vi "Pair Nodes.vi"(8 "error in (no error)":errorcluster, 10 "Node UID to Pair":string, 11 "E2E editor node in":refnum<data-value>) -> (0 "error out":errorcluster, 3 "E2E editor node out":refnum<data-value>)   [LabVIEW 2015, in "E2E Tag Exchange editor node.lvclass"]
uses:
  E2E Tag Exchange editor node.lvclass
  Node LUT/Command.ctl
  Node LUT/Node LUT.lvlib
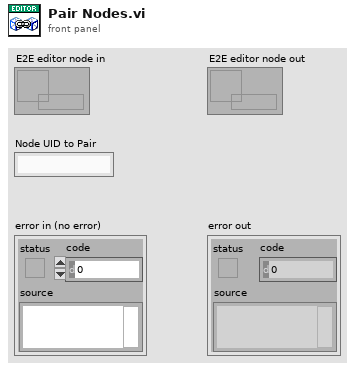
[diagram p1: front panel]
types:
  T1 = typedef "Node LUT.lvlib/Command.ctl" = enum16{"Initialize", "Add Node", "Remove Node", "Node Ref from UID", "List Nodes"}
  T2 = typedef "NISE_CEF_Node.lvclass/NodeRef.ctl" = refnum<data-value>
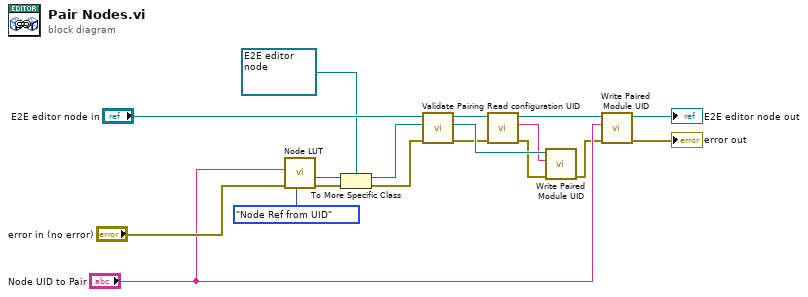
[diagram p0: block diagram]
diagram:
  n1 = call "Node LUT.vi"("Command"=Command."Node Ref from UID", "error in"="error in (no error)", "UID"="Node UID to Pair") -> ("error out"=w14:errorcluster, "node ref"=w15:T2)  [unwired: 5 in, 2 out]
  n2 = To More Specific Class(target class=refnum<data-value> refnum, reference=w15, error in=w14) -> (specific class reference=w12:refnum<data-value>, error out=w11:errorcluster)
  n3 = call "Validate Pairing.vi"("error in (no error)"=w11, "E2E node 2"=w12, "E2E node 1"="E2E editor node in") -> ("error out"=w4:errorcluster, "E2E node 2 out"=w5:refnum<data-value>, "E2E node 1 out"=w7:refnum<data-value>)  [unwired: 6 in]
  n4 = call "Read configuration UID.vi"("error in (no error)"=w4, "E2E editor node in"=w7) -> ("error out"=w3:errorcluster, "Module UID"=w2:string, "E2E editor node out"=w6:refnum<data-value>)  [unwired: 7 in]
  n5 = call "Write Paired Module UID.vi"("error in (no error)"=w3, "Paired Module UID"=w2, "E2E editor node in"=w5) -> ("error out"=w1:errorcluster)  [unwired: 7 in, 1 out]
  n6 = call "Write Paired Module UID.vi"("error in (no error)"=w1, "Paired Module UID"="Node UID to Pair", "E2E editor node in"=w6) -> ("error out"=→"error out":errorcluster, "E2E editor node out"=→"E2E editor node out":refnum<data-value>)  [unwired: 7 in]
